vi "HXG2_Air Psychs.vi"(0 "Air Out Avg (°F)":dbl, 1 "Air In Avg (°F)":dbl, 5 "Air flow (scfm)":dbl, 7 "Patm (psia)":dbl, 9 "Nozzle In Hum (%)":dbl, 11 "error in (no error)":errorcluster, 12 "dP Product (inWC)":dbl) -> (4 "Air rho (lbm/ft³)":dbl, 6 "Air Q (BTU/hr)":dbl, 8 "Air Cp (BTU/lb)":dbl, 10 "Air Q (W)":dbl, 14 "acfm":dbl, 15 "error out":errorcluster)   [LabVIEW 2010]
doc: "This VI will comlplete psychrometric calculations and output density of air and complete the calculation to figure out the heat load on the air side and finalizes with the conversion from SCFM to ACFM. The ACFM calculation is documented at the bottom of the block diagram."
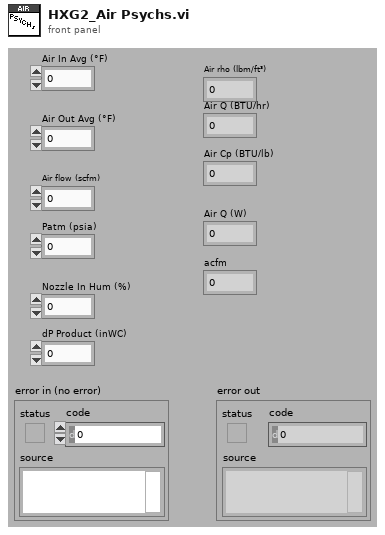
[diagram p1: front panel]
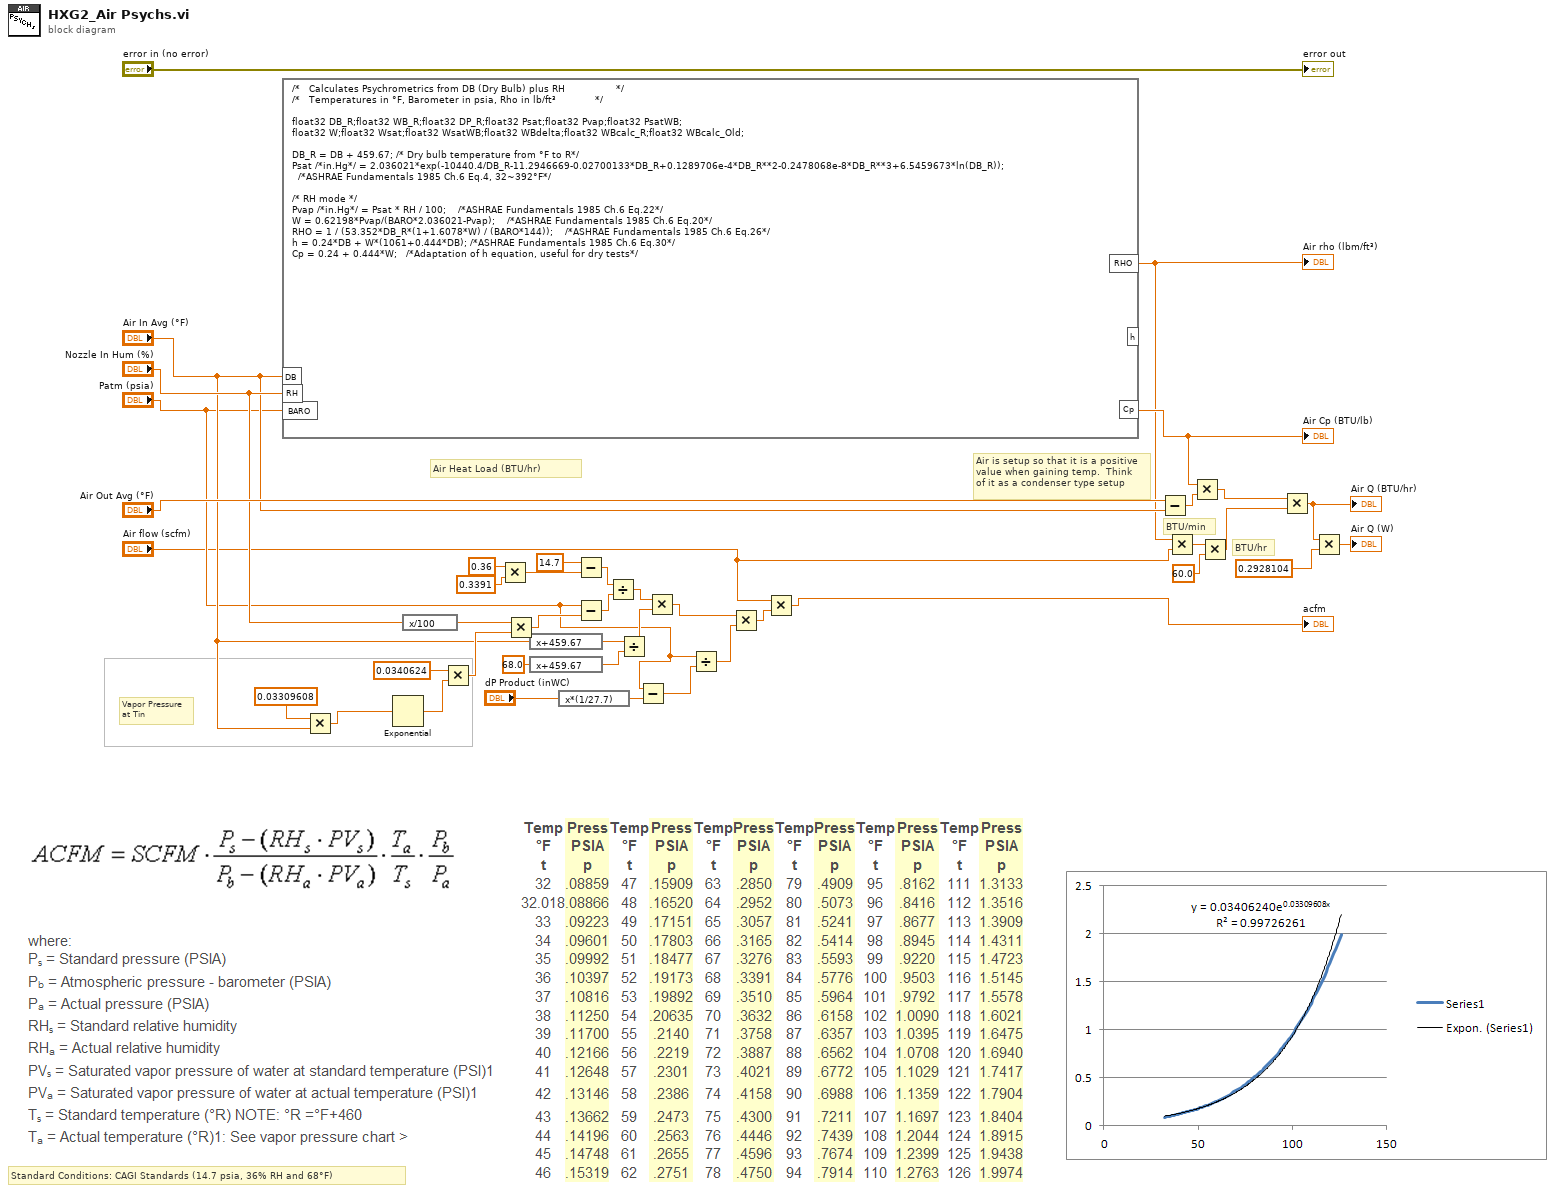
[diagram p0: block diagram]
diagram:
  # "Air is setup so that it is a positive\nvalue when gaining temp.  Think\nof it as a condenser type setup"
  # "BTU/hr"
  # "BTU/min"
  # "Vapor Pressure\nat Tin"
  # "Standard Conditions: CAGI Standards (14.7 psia, 36% RH and 68°F)"
  # "Air Heat Load (BTU/hr)"
  n1 = formula code="/*   Calculates Psychrometrics from DB (Dry Bulb) plus RH                 */\n/*   Temperatures in °F, Barometer in psia, Rho in lb/ft³             */\n\nfloat32 DB_R;float32 WB_R;float32 DP_R;float32 Psat;float32 Pvap;float32 PsatWB;\nfloat32 W;float32 Wsat;float32 WsatWB;float32 WBdelta;float32 WBcalc_R;float32 WBcalc_Old;\n\nDB_R = DB + 459.67; /* Dry bulb temperature from °F to R*/\nPsat /*in.Hg*/ = 2.036021*exp(-10440.4/DB_R-11.2946669-0.02700133*DB_R+0.1289706e-4*DB_R**2-0.2478068e-8*DB_R**3+6.5459673*ln(DB_R));  \n  /*ASHRAE Fundamentals 1985 Ch.6 Eq.4, 32~392°F*/\n\n/* RH mode */\nPvap /*in.Hg*/ = Psat * RH / 100;    /*ASHRAE Fundamentals 1985 Ch.6 Eq.22*/\nW = 0.62198*Pvap/(BARO*2.036021-Pvap);    /*ASHRAE Fundamentals 1985 Ch.6 Eq.20*/\nRHO = 1 / (53.352*DB_R*(1+1.6078*W) / (BARO*144));    /*ASHRAE Fundamentals 1985 Ch.6 Eq.26*/\nh = 0.24*DB + W*(1061+0.444*DB); /*ASHRAE Fundamentals 1985 Ch.6 Eq.30*/\nCp = 0.24 + 0.444*W;   /*Adaptation of h equation, useful for dry tests*/"("DB"="Air In Avg (°F)", "BARO"="Patm (psia)", "RH"="Nozzle In Hum (%)") -> ("RHO"=w5:dbl, "Cp"=w38:dbl)  [unwired: 1 out]
  "Air Cp (BTU/lb)" <- w38
  "Air rho (lbm/ft³)" <- w5
  n2 = Multiply(x=0.03309608, y="Air In Avg (°F)") -> (x*y=w25:dbl)
  n3 = Exponential(1:w25) -> (0:w24:dbl)
  n4 = expression code="x/100"("Nozzle In Hum (%)") -> (w7:dbl)
  n5 = Multiply(x=0.0340624, y=w24) -> (x*y=w23:dbl)
  n6 = Multiply(x=0.36, y=0.3391 ("x")) -> (x*y=w31:dbl)
  n7 = Multiply(x=w7, y=w23) -> (x*y=w22:dbl)
  n8 = expression code="x+459.67"("Air In Avg (°F)") -> (w17:dbl)
  n9 = expression code="x+459.67"(68.0 ("x")) -> (w16:dbl)
  n10 = expression code="x*(1/27.7)"("dP Product (inWC)") -> (w10:dbl)
  n11 = Subtract(x=14.7, y=w31) -> (x-y=w21:dbl)
  n12 = Subtract(x="Patm (psia)", y=w22) -> (x-y=w20:dbl)
  n13 = Divide(x=w21, y=w20) -> (x/y=w19:dbl)
  n14 = Divide(x=w17, y=w16) -> (x/y=w14:dbl)
  n15 = Subtract(x="Patm (psia)", y=w10) -> (x-y=w8:dbl)
  n16 = Multiply(x=w19, y=w14) -> (x*y=w13:dbl)
  n17 = Divide(x="Patm (psia)", y=w8) -> (x/y=w12:dbl)
  n18 = Multiply(x=w13, y=w12) -> (x*y=w6:dbl)
  n19 = Multiply(x="Air flow (scfm)", y=w6) -> (x*y=→"acfm":dbl)
  n20 = Subtract(x="Air Out Avg (°F)", y="Air In Avg (°F)") -> (x-y=w39:dbl)
  n21 = Multiply(x=w5, y="Air flow (scfm)") -> (x*y=w33:dbl)
  n22 = Multiply(x=w38, y=w39) -> (x*y=w37:dbl)
  n23 = Multiply(x=w33, y=60.0) -> (x*y=w4:dbl)
  n24 = Multiply(x=w37, y=w4) -> (x*y=w36:dbl)
  "Air Q (BTU/hr)" <- w36
  n25 = Multiply(x=w36, y=0.2928104) -> (x*y=→"Air Q (W)":dbl)
  "error out" <- "error in (no error)"
